vi "Configure Thermocouple.vi"(0 "VISA resource name":refnum<visa-resource-name>, 1 "Thermocouple Type (0: J)":u16(ring) items=["E", "N", "B", "C", "K", "J", "R", "S", "T"], 2 "R-Junction Type (0: Simulated)":u16(ring) items=["Simulated", "Real"], 3 "Function":i32(ring) items=["Primary", "Secondary"], 5 "error in (no error)":errorcluster, 6 "Simulated Temperature (23.00 deg)":dbl=23.0 format="%_4f", 7 "Digital Filter (0: Off)":u16(ring) items=["Off", "Moving Filter", "Repeating Filter"], 8 "Temperature Units (0: Celsius)":u16(ring) items=["Celsius", "Fahrenheit", "Kelvin"], 9 "Digital Filter Readings (10)":i32=10) -> (14 "VISA resource name out":refnum<visa-resource-name>, 19 "error out":errorcluster)   [LabVIEW 2024, in "Keithley 2100 Series.lvlib"]
doc: "This VI configures the thermocouple type and settings."
uses:
  Keithley 2100 Series.lvlib
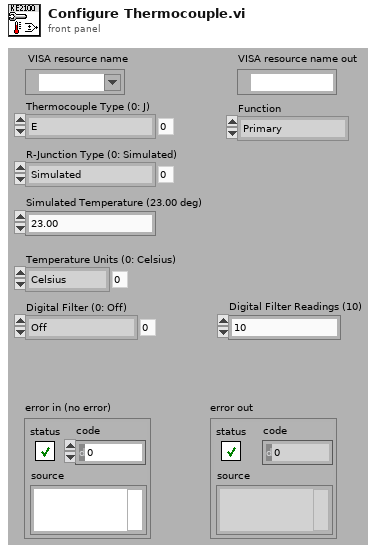
[diagram p1: front panel]
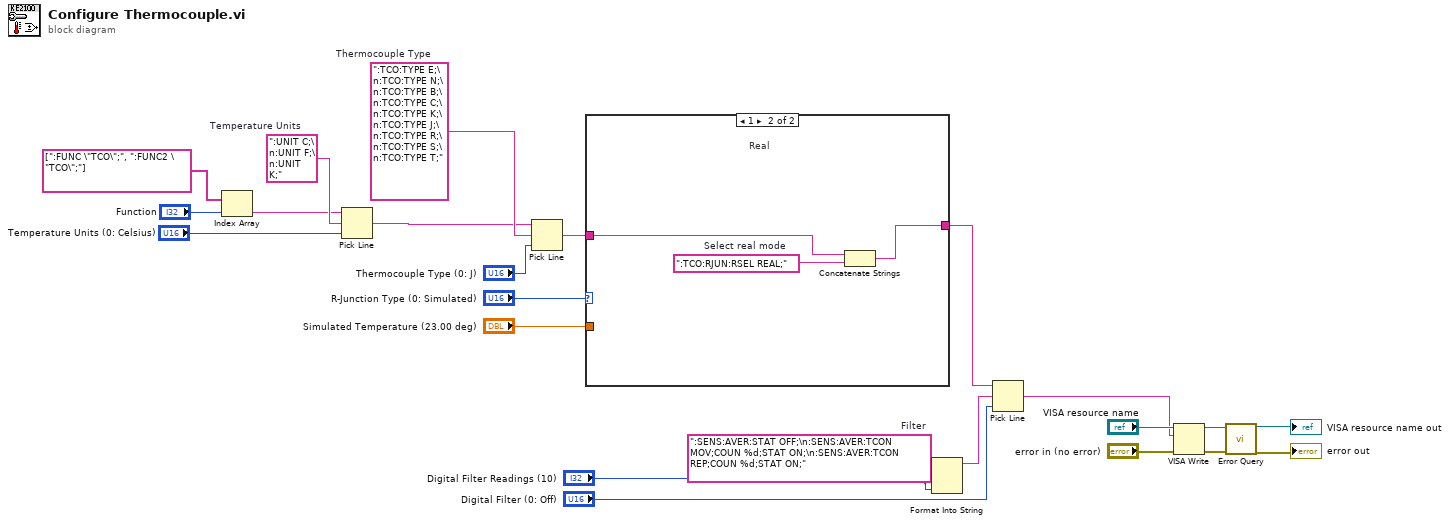
[diagram p0: block diagram]
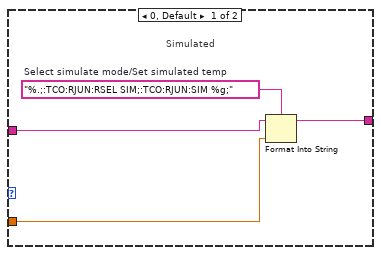
[diagram p2: hidden frame]
diagram:
  w10 = ":SENS:AVER:STAT OFF;\n:SENS:AVER:TCON MOV;COUN %d;STAT ON;\n:SENS:AVER:TCON REP;COUN %d;STAT ON;"  # Filter
  w12 = ":UNIT C;\n:UNIT F;\n:UNIT K;"  # Temperature Units
  w21 = ":TCO:TYPE E;\n:TCO:TYPE N;\n:TCO:TYPE B;\n:TCO:TYPE C;\n:TCO:TYPE K;\n:TCO:TYPE J;\n:TCO:TYPE R;\n:TCO:TYPE S;\n:TCO:TYPE T;"  # Thermocouple Type
  n1 = Index Array(array=string[] [":FUNC \"TCO\";", ":FUNC2 \"TCO\";"], index="Function") -> (element=w1:string)
  n2 = Pick Line(string ("")=w1, multi-line string=w12, line index="Temperature Units (0: Celsius)") -> (output string=w4:string)
  n3 = Pick Line(string ("")=w4, multi-line string=w21, line index="Thermocouple Type (0: J)") -> (output string=w17:string)
  n4 = case shown="1" "R-Junction Type (0: Simulated)" {
    tunnel: "Simulated Temperature (23.00 deg)" -> [w25 _]
    tunnel: w17 -> [w27 w30]
    tunnel: [w24 w28] -> w6
    frame 0, Default {
      w26 = "%.;:TCO:RJUN:RSEL SIM;:TCO:RJUN:SIM %g;"  # Select simulate mode/Set simulated temp
      # "Simulated"
      n5 = Format Into String(format string=w26, initial string=w27, w25) -> (resulting string=w24:string)  [unwired: 1 in, 1 out]
    }
    frame 1 {
      w29 = ":TCO:RJUN:RSEL REAL;"  # Select real mode
      # "Real"
      n6 = Concatenate Strings(w30, w29) -> (w28:string)
    }
  }
  n7 = Format Into String(format string=w10, "Digital Filter Readings (10)", "Digital Filter Readings (10)") -> (resulting string=w9:string)  [unwired: 2 in, 1 out]
  n8 = Pick Line(string ("")=w6, multi-line string=w9, line index="Digital Filter (0: Off)") -> (output string=w5:string)
  n9 = VISA Write(VISA resource name="VISA resource name", write buffer=w5, error in (no error)="error in (no error)") -> (VISA resource name out=w16:refnum<visa-resource-name>, error out=w14:errorcluster)  [unwired: 1 out]
  n10 = call "Error Query.vi"("VISA resource name"=w16, "error in (no error)"=w14) -> ("VISA resource name out"=→"VISA resource name out":refnum<visa-resource-name>, "error out"=→"error out":errorcluster)  [unwired: 14 in, 2 out]
